vi "回貨明細.vi"() -> ()   [LabVIEW 2012]
uses:
  <vilib>/Utility/NIReport.llb/NI_report.lvclass
  Global1.vi
  <vilib>/addons/database/Connection.llb/DB Tools Open Connec (Path).vi
  <vilib>/addons/_office/excel.llb/Excel Get Data (str).vi
  <vilib>/Utility/NIReport.llb/Excel/NI_Excel.lvclass
  <vilib>/addons/_office/NI_ReportGenerationToolkit.lvlib
  <vilib>/addons/database/NI_Database_API.lvlib
panel:
  in  "path":path=path "O:/Monitor/回貨明細/回貨明細_1031.xls"
  in  "start (0, 0)":cluster{"start row":i32, "start column":i32}
  out "error out 4":errorcluster
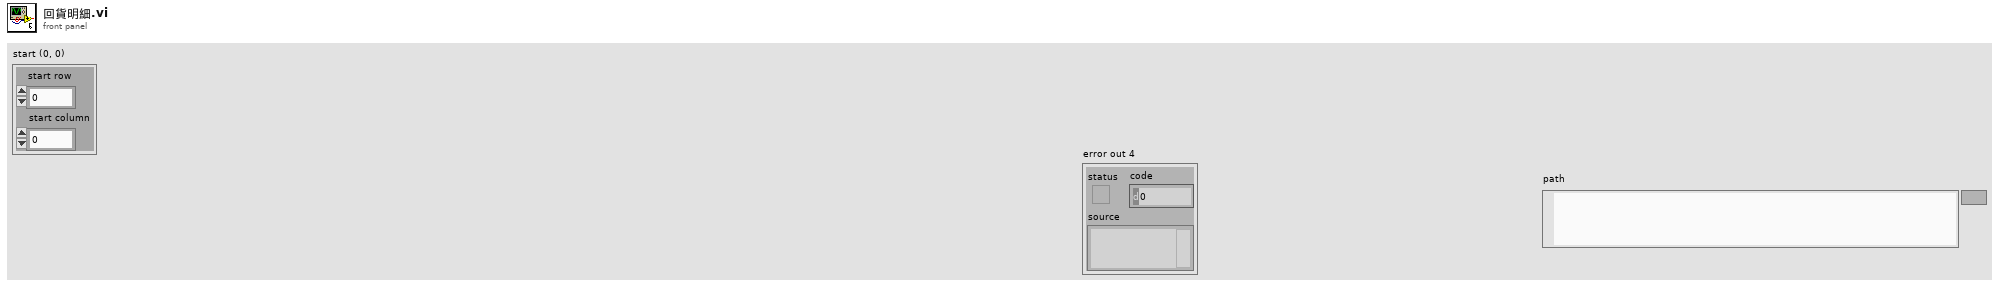
[diagram p1: front panel]
types:
  T1 = enum16{"Standard Report", "HTML", "Word", "Excel"}
  T2 = typedef "NI_Database_API.lvlib/Conn ObjectReference.ctl" = refnum<k1>
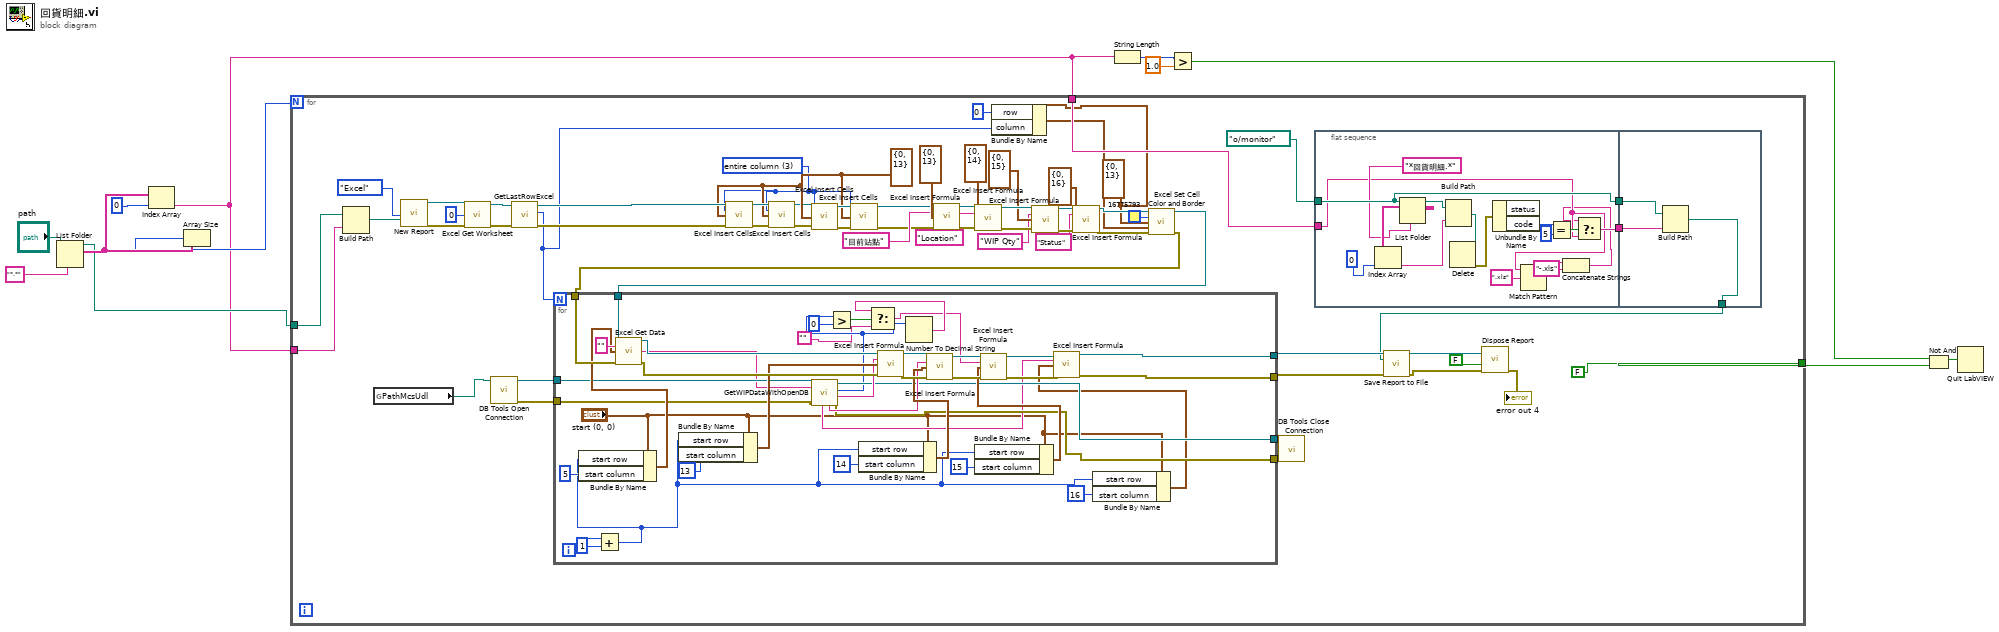
[diagram p0: block diagram]
diagram:
  n1 = List Folder(path="path", pattern="*.*") -> (path out=w4:path, filenames=w7:string[])  [unwired: 2 in, 2 out]
  n2 = Index Array "Index Array"(array=w7, index=0) -> (element=w3:string)
  n3 = Array Size(array=w7) -> (size(s)=w5:i32)
  n4 = for {
    N: w5 -> [_]
    tunnel: w4 -> [w73]
    tunnel: w3 -> [w72]
    tunnel: w3 -> [w70]
    tunnel: [FALSE] -> w8
    w16 = cluster{"row":i32, "column":i32} {"row"=0, "column"=13} ("start (-1, -1)")
    w39 = cluster{"row":i32, "column":i32} {"row"=0, "column"=13} ("start (0, 0)")
    w36 = u16 3 items=["shift cells right", "shift cells down", "entire row", "entire column"] ("mode (entire row)")
    n5 = Build Path(base path=w73, name or relative path=w72) -> (appended path=w71:path)
    n6 = global read "Global1.vi" "PathMcsUdl"() -> (w62:path)
    n7 = call <vilib>:"New Report.vi"("report type"=T1."Excel" ("Report Type"), "template (empty)"=w71) -> ("report out"=w68:refnum<class "NI_report.lvclass">, "error out"=w67:errorcluster)  [unwired: 12 in]
    n8 = call <vilib>:"Excel Get Worksheet.vi"("report in"=w68, "worksheet index (0)"=0, "error in (no error)"=w67) -> ("report out"=w45:refnum<class "NI_report.lvclass">, "error out"=w44:errorcluster)  [unwired: 11 in]
    n9 = call-poly <vilib>:"DB Tools Open Connection.vi"("connection information"=w62) -> ("error out"=w60:errorcluster, "connection reference"=w61:T2)  [unwired: 7 in]
    n10 = call "GetLastRowExcel.vi"("error in (no error)"=w44, "report in"=w45) -> ("error out"=w43:errorcluster, "row"=w14:i32, "report out"=w42:refnum<class "NI_report.lvclass">)  [unwired: 7 in]
    n11 = call <vilib>:"Excel Insert Cells.vi"("report in"=w42, "mode (entire row)"=w36, "start (0, 0)"=w39, "error in (no error)"=w43) -> ("report out"=w41:refnum<class "NI_report.lvclass">, "error out"=w40:errorcluster)  [unwired: 10 in]
    n12 = call <vilib>:"Excel Insert Cells.vi"("report in"=w41, "mode (entire row)"=w36, "start (0, 0)"=w39, "error in (no error)"=w40) -> ("report out"=w38:refnum<class "NI_report.lvclass">, "error out"=w37:errorcluster)  [unwired: 10 in]
    n13 = call <vilib>:"Excel Insert Cells.vi"("report in"=w38, "mode (entire row)"=w36, "start (0, 0)"=w39, "error in (no error)"=w37) -> ("report out"=w66:refnum<class "NI_report.lvclass">, "error out"=w65:errorcluster)  [unwired: 10 in]
    n14 = call <vilib>:"Excel Insert Cells.vi"("report in"=w66, "mode (entire row)"=w36, "start (0, 0)"=w39, "error in (no error)"=w65) -> ("report out"=w23:refnum<class "NI_report.lvclass">, "error out"=w22:errorcluster)  [unwired: 10 in]
    n15 = call <vilib>:"Excel Insert Formula.vi"("report in"=w23, "formula"="目前站點", "start (0, 0)"=cluster{"row":i32, "column":i32} {"row"=0, "column"=13}, "error in (no error)"=w22) -> ("report out"=w59:refnum<class "NI_report.lvclass">, "error out"=w57:errorcluster)  [unwired: 10 in]
    n16 = call <vilib>:"Excel Insert Formula.vi"("report in"=w59, "formula"="Location", "start (0, 0)"=cluster{"row":i32, "column":i32} {"row"=0, "column"=14}, "error in (no error)"=w57) -> ("report out"=w58:refnum<class "NI_report.lvclass">, "error out"=w56:errorcluster)  [unwired: 10 in]
    n17 = Bundle By Name(cluster=w16, "row"=0, "column"=w14) -> (w17:cluster{"row":i32, "column":i32})
    n18 = call <vilib>:"Excel Insert Formula.vi"("report in"=w58, "formula"="WIP Qty", "start (0, 0)"=cluster{"row":i32, "column":i32} {"row"=0, "column"=15}, "error in (no error)"=w56) -> ("report out"=w35:refnum<class "NI_report.lvclass">, "error out"=w34:errorcluster)  [unwired: 10 in]
    n19 = call <vilib>:"Excel Insert Formula.vi"("report in"=w35, "formula"="Status", "start (0, 0)"=cluster{"row":i32, "column":i32} {"row"=0, "column"=16}, "error in (no error)"=w34) -> ("report out"=w21:refnum<class "NI_report.lvclass">, "error out"=w20:errorcluster)  [unwired: 10 in]
    n20 = call <vilib>:"Excel Set Cell Color and Border.vi"("report in"=w21, "background color (w)"=u32 16775793, "start (-1, -1)"=w16, "end (-1, -1)"=w17, "error in (no error)"=w20) -> ("report out"=w19:refnum<class "NI_report.lvclass">, "error out"=w18:errorcluster)  [unwired: 9 in]
    n21 = for {
      N: w14 -> [_]
      tunnel: w19 -> [w134]
      tunnel: w18 -> [w133]
      tunnel: [w94] -> w46
      tunnel: [w115] -> w64
      tunnel: [w114] -> w63
      tunnel: w61 -> [w113]
      tunnel: w60 -> [w112]
      tunnel: [w95] -> w32
      i -> [w105]
      n22 = Add(x=w105, y=1) -> (x+y=w98:i32)
      n23 = Bundle By Name(cluster="start (0, 0)", "start row"=w98, "start column"=5) -> (w128:cluster{"start row":i32, "start column":i32})
      n24 = call-poly <vilib>:"Excel Get Data.vi"("report in"=w134, "data type"="", "start (0, 0)"=w128, "error in (no error)"=w133) -> ("report out"=w131:refnum<class "NI_report.lvclass">, "data"=w96:string, "error out"=w130:errorcluster)  [unwired: 9 in]
      n25 = Bundle By Name(cluster="start (0, 0)", "start row"=w98, "start column"=13) -> (w126:cluster{"start row":i32, "start column":i32})
      n26 = call "GetWIPDataWithOpenDB.vi"("error in (no error)"=w112, "Lotno"=w96, "connection reference"=w113) -> ("error out"=w114:errorcluster, "step"=w117:string, "data"=w110:i32, "connection reference 2"=w115:T2, "location"=w116:string, "status"=w99:string)  [unwired: 3 in]
      n27 = Greater?(x=w110, y=0) -> (0:w108:bool)
      n28 = Bundle By Name(cluster="start (0, 0)", "start row"=w98, "start column"=14) -> (w118:cluster{"start row":i32, "start column":i32})
      n29 = call <vilib>:"Excel Insert Formula.vi"("report in"=w131, "formula"=w117, "start (0, 0)"=w126, "error in (no error)"=w130) -> ("report out"=w123:refnum<class "NI_report.lvclass">, "error out"=w120:errorcluster)  [unwired: 10 in]
      n30 = Number To Decimal String(number=w110) -> (decimal integer string=w109:string)  [unwired: 1 in]
      n31 = Select(t=w109, s=w108, f="") -> (s? t:f=w106:string)
      n32 = call <vilib>:"Excel Insert Formula.vi"("report in"=w123, "formula"=w116, "start (0, 0)"=w118, "error in (no error)"=w120) -> ("report out"=w122:refnum<class "NI_report.lvclass">, "error out"=w121:errorcluster)  [unwired: 10 in]
      n33 = Bundle By Name(cluster="start (0, 0)", "start row"=w98, "start column"=15) -> (w119:cluster{"start row":i32, "start column":i32})
      n34 = call <vilib>:"Excel Insert Formula.vi"("report in"=w122, "formula"=w106, "start (0, 0)"=w119, "error in (no error)"=w121) -> ("report out"=w102:refnum<class "NI_report.lvclass">, "error out"=w101:errorcluster)  [unwired: 10 in]
      n35 = Bundle By Name(cluster="start (0, 0)", "start row"=w98, "start column"=16) -> (w100:cluster{"start row":i32, "start column":i32})
      n36 = call <vilib>:"Excel Insert Formula.vi"("report in"=w102, "formula"=w99, "start (0, 0)"=w100, "error in (no error)"=w101) -> ("report out"=w95:refnum<class "NI_report.lvclass">, "error out"=w94:errorcluster)  [unwired: 10 in]
    }
    n37 = call <vilib>:"DB Tools Close Connection.vi"("error in (no error)"=w63, "connection reference"=w64) -> ()  [unwired: 5 in, 1 out]
    n38 = flat-sequence {
      tunnel: path "o:/monitor" ("base path") -> [w86]
      tunnel: [w86] -> w26
      tunnel: w70 -> [w75]
      tunnel: [w76] -> w25
      tunnel: w26 -> [w93]
      tunnel: [w92] -> w28
      tunnel: w25 -> [w91]
      frame #0 {
        n39 = List Folder(path=w86, pattern="*回貨明細.*") -> (path out=w88:path, filenames=w90:string[])  [unwired: 2 in, 2 out]
        n40 = Index Array(array=w90, index=0) -> (element=w87:string)
        n41 = Build Path(base path=w88, name or relative path=w87) -> (appended path=w84:path)
        n42 = Delete(path (use dialog)=w84) -> (error out=w83:errorcluster)  [unwired: 4 in, 2 out]
        n43 = Unbundle By Name(w83) -> ("code"=w82:i32)  [unwired: 1 out]
        n44 = Match Pattern(string=w75, regular expression=".xls") -> (match substring=w78:string)  [unwired: 1 in, 3 out]
        n45 = Equal?(x=w82, y=5) -> (x = y?=w80:bool)
        n46 = Concatenate Strings(w78, "-.xls" ("string")) -> (w74:string)
        n47 = Select(t=w74, s=w80, f=w75) -> (s? t:f=w76:string)
      }
      frame #1 {
        n48 = Build Path(base path=w93, name or relative path=w91) -> (appended path=w92:path)
      }
    }
    n49 = call-dynamic "Save Report to File.vi"("report in"=w32, "report file path"=w28, "error in (no error)"=w46) -> ("report out"=w31:refnum<class "NI_report.lvclass">, "error out"=w47:errorcluster)  [unwired: 11 in]
    n50 = call-dynamic "Dispose Report.vi"("report in"=w31, "save changes? (F)"=FALSE, "error in (no error)"=w47) -> ("error out"=→"error out 4":errorcluster)  [unwired: 12 in]
  }
  n51 = String Length(string=w3) -> (length=w11:i32)
  n52 = Greater?(x=w11, y=1.0) -> (0:w9:bool)
  n53 = Not And(1:w8, 2:w9) -> (0:w10:bool)
  n54 = Quit LabVIEW(quit? (T)=w10) -> ()
